vi "Kursovaya.vi"() -> ()   [LabVIEW 2013]
panel:
  in  "stop":bool
  out "return count":u32
  in  "Write":string
  out "Read Data":string
  in  "byte count":u32
  in  "VISA resource name":refnum<visa-resource-name>
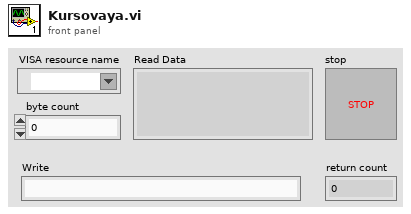
[diagram p1: front panel]
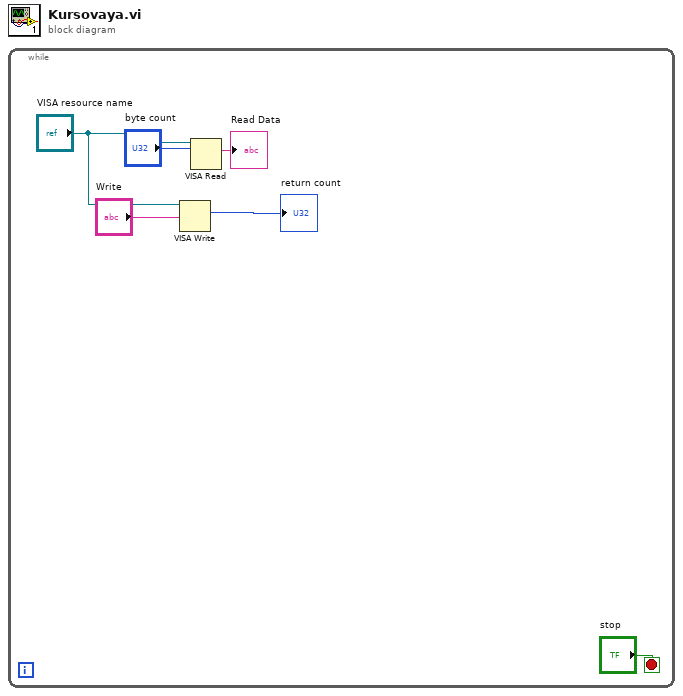
[diagram p0: block diagram]
diagram:
  n1 = while {
    stop <- "stop" stop-if-true
    n2 = VISA Write(VISA resource name="VISA resource name", write buffer="Write") -> (return count=→"return count":u32)  [unwired: 1 in, 2 out]
    n3 = VISA Read(VISA resource name="VISA resource name", byte count="byte count") -> (read buffer=→"Read Data":string)  [unwired: 1 in, 3 out]
  }
